vi "Ex2_ServoControl2.vi"() -> ()   [LabVIEW 2024]
panel:
  in  "Boolean":bool
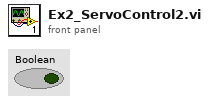
[diagram p1: front panel]
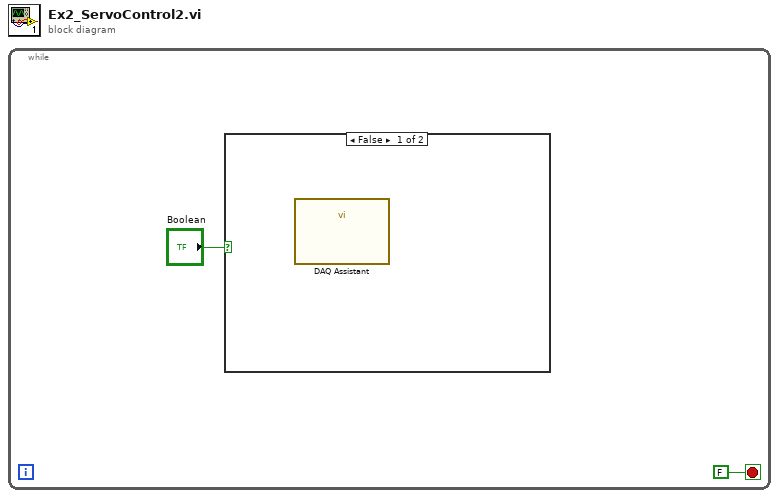
[diagram p0: block diagram]
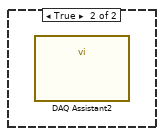
[diagram p2: hidden frame]
diagram:
  n1 = while {
    stop <- FALSE stop-if-true
    n2 = case shown="False" "Boolean" {
      frame False {
        n3 = call "DAQ Assistant"() -> ()  [unwired: 18 in, 2 out]
      }
      frame True {
        n4 = call "DAQ Assistant2"() -> ()  [unwired: 18 in, 2 out]
      }
    }
  }
